vi "George_Illumination.vi"(0 "File Path":path=path "C:/Test_Data/George_Illumination/L127Capture Image_.bmp", 7 "error in":errorcluster) -> (20 "Line Profile (Illumination Line Profile [Horizantal])":cluster{"x0":sgl, "dx":sgl, "Pixels Line":sgl[]}={"x0"=0.0, "dx"=1.0, "Pixels Line"=[0.0]} {"Pixels Line" format="%.2f"; "dx" format="%.2f"; "x0" format="%.2f"}, 21 "ROI Pixel Statistics (Illumination Line Profile [Horizantal])":T2 {"Min" format="%.2f"; "Std Dev" format="%.2f"; "Mean" format="%.2f"; "Max" format="%.2f"}, 22 "Line Profile (Illumination Line Profile [Vertical])":cluster{"x0":sgl, "dx":sgl, "Pixels Line":sgl[]}={"x0"=0.0, "dx"=1.0, "Pixels Line"=[0.0]} {"Pixels Line" format="%.2f"; "dx" format="%.2f"; "x0" format="%.2f"}, 23 "ROI Pixel Statistics (Illumination Line Profile [Vertical])":T2 {"Min" format="%.2f"; "Std Dev" format="%.2f"; "Mean" format="%.2f"; "Max" format="%.2f"}, 27 "error out":errorcluster={"status"=TRUE, "code"=-1074396120, "source"="IMAQ ROIProfile\n  "})   [LabVIEW 2014]
uses:
  <vilib>/vision/NI_Vision_Development_Module.lvlib
panel:
  out "Image Out":T1(plugin-control)
  out "Line Profile Graph 2":cluster{"x0":sgl, "dx":sgl, "Pixels Line":sgl[]}(graph)={"x0"=0.0, "dx"=1.0, "Pixels Line"=[0.0]} caption="Line Profile"
  out "Line Profile Graph":cluster{"x0":sgl, "dx":sgl, "Pixels Line":sgl[]}(graph)={"x0"=0.0, "dx"=1.0, "Pixels Line"=[0.0]} caption="Line Profile"
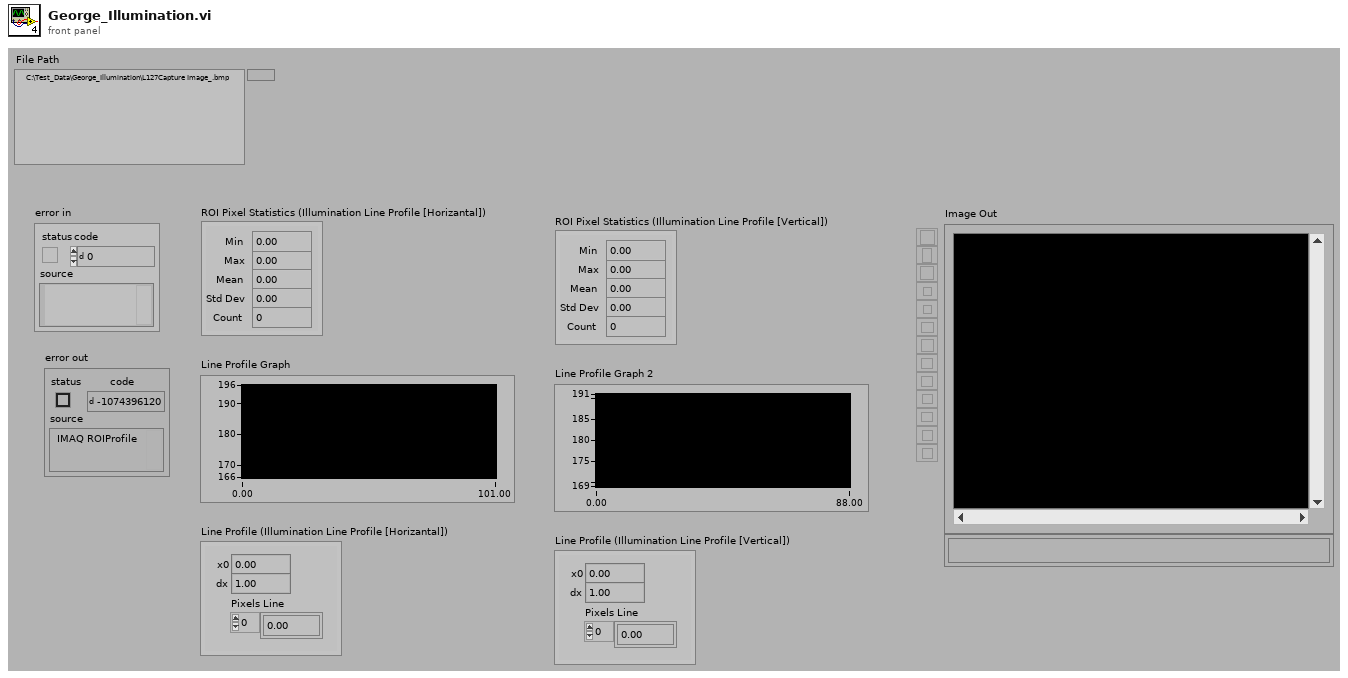
[diagram p1: front panel]
types:
  T1 = typedef "IMAQ Image.ctl" = refnum<image>
  T2 = cluster{"Min":sgl, "Max":sgl, "Mean":sgl, "Std Dev":sgl, "Count":i32}
  T3 = cluster{"Global Rectangle":i32[], "Contours":cluster{"ID":enum32{"External", "Internal"}, "Type":u32, "Coordinates":i32[]}[]}
  T4 = cluster{"Origin":cluster{"X":sgl, "Y":sgl}, "Angle (deg)":sgl, "Axis Reference":u32}
  T5 = enum16{"Reset", "Update Coordinate System", "Get Coordinate System"}
  T6 = enum16{"Horizontal Motion", "Vertical Motion", "Horizontal and Vertical Motion", "Horizontal, Vertical and Angular Motion"}
  T7 = typedef "Image Type" = u32
  T8 = typedef "IMAQ Coordinate System" = cluster{"Reference System":cluster{"Origin":cluster{"X":sgl, "Y":sgl}, "Angle (deg)":sgl, "Axis Reference":u32}, "Measurement System":cluster{"Origin":cluster{"X":sgl, "Y":sgl}, "Angle (deg)":sgl, "Axis Reference":u32}}
  T9 = typedef "ROI Descriptor" = cluster{"Global Rectangle":i32[], "Contours":cluster{"ID":enum32{"External", "Internal"}, "Type":u32, "Coordinates":i32[]}[]}
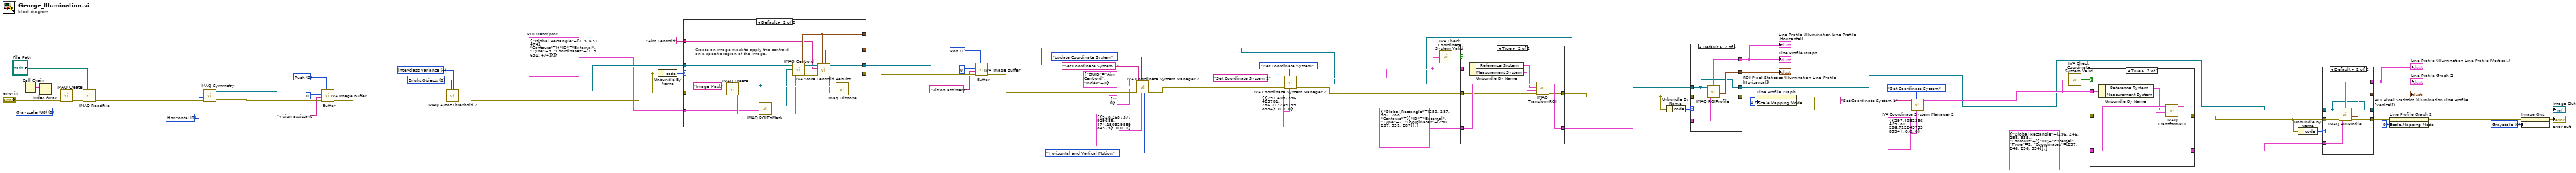
[diagram p0: block diagram]
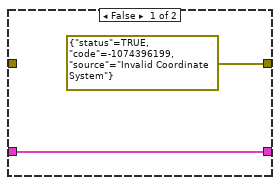
[diagram p3: hidden frame]
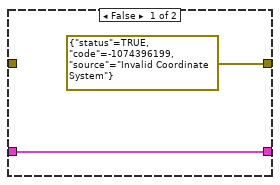
[diagram p5: hidden frame]
diagram:
  w3 = u32 0 items=["Grayscale", "Binary", "Gradient", "Rainbow", "Temperature", "User Defined"] ("Palette")
  w46 = u16 1 items=["Push", "Pop", "Reset"] ("Function")
  w51 = T3 {"Global Rectangle"=[7, 5, 631, 474], "Contours"=[{"ID"=enum."External", "Type"=3, "Coordinates"=[7, 5, 631, 474]}]}  # ROI Descriptor
  w54 = 4 items=["clustering", "entropy", "metric", "moments", "inter-class variance"] ("Method")
  w55 = u32 0 items=["Bright Objects", "Dark Objects"] ("Look For")
  w60 = u16 0 items=["Push", "Pop", "Reset"] ("Function")
  w63 = u32 0 items=["Horizontal", "Vertical", "Central", "1st Diagonal", "2nd Diagonal"] ("Type of Symmetry")
  w66 = T7 0 items=["Grayscale (U8)", "Grayscale (I16)", "Grayscale (SGL)", "Complex (CSG)", "RGB (U32)", "HSL (U32)", "RGB (U64)", "Grayscale (U16)"] ("Image Type")
  # "Buffer"
  # "Buffer"
  n1 = Call Chain() -> (call chain=w68:string[])
  n2 = Index Array(array=w68) -> (element=w67:string)  [unwired: 1 in]
  n3 = call "IMAQ Create"("Image Name"=w67, "Image Type"=w66, "error in (no error)"="error in") -> ("New Image"=w71:T1, "error out"=w70:errorcluster)  [unwired: 1 in, 1 out]
  n4 = call "IMAQ ReadFile"("File Path"="File Path", "error in (no error)"=w70, "Image"=w71) -> ("error out"=w72:errorcluster, "Image Out"=w65:T1)  [unwired: 2 in, 5 out]
  n5 = call "IMAQ Symmetry"("error in (no error)"=w72, "Type of Symmetry"=w63, "Image Src"=w65) -> ("error out"=w64:errorcluster, "Image Dst Out"=w62:T1)  [unwired: 1 in, 1 out]
  n6 = call <vilib>:"IVA Image Buffer.vi"("Function"=w60, "error in (no error)"=w64, "Prefix"="vision assistant", "Buffer #"=0, "Image In"=w62) -> ("error out"=w61:errorcluster, "Image Out"=w57:T1)  [unwired: 5 out]
  n7 = call "IMAQ AutoBThreshold 2"("Image Src"=w57, "Look For (Bright Objects)"=w55, "Method (clustering)"=w54, "error in (no error)"=w61) -> ("Image Dst Out"=w52:T1, "error out"=w56:errorcluster)  [unwired: 4 in, 6 out]
  n8 = Unbundle By Name(w56) -> ("code"=w49:i32)
  n9 = case shown="Default" w49 {
    tunnel: w56 -> [_ w84]
    tunnel: [_ w83] -> w53
    tunnel: w52 -> [w73 w81]
    tunnel: [w73 w80] -> w48
    tunnel: [_ w79] -> _
    tunnel: [_ w78] -> _
    tunnel: w51 -> [_ w77]
    tunnel: "Aim Centroid" ("Step Name") -> [_ w74]
    frame -1074396199, -1074396198 {
      # "Discard Coordinate System Error"
    }
    frame Default {
      # "Create an image mask to apply the centroid\non a specific region of the image."
      n10 = call "IMAQ Create"("Image Name"="Image Mask", "error in (no error)"=w84) -> ("New Image"=w87:T1, "error out"=w86:errorcluster)  [unwired: 2 in, 1 out]
      n11 = call "IMAQ ROIToMask"("error in (no error)"=w86, "ROI Descriptor"=w77, "Image"=w87) -> ("error out"=w82:errorcluster, "Image Out"=w85:T1)  [unwired: 2 in, 2 out]
      n12 = call "IMAQ Centroid"("error in (no error)"=w82, "Image Mask"=w85, "Image"=w81) -> ("error out"=w76:errorcluster, "Centroid"=w79:cluster{"X Centroid":sgl, "Y Centroid":sgl})  [unwired: 1 out]
      n13 = call <vilib>:"IVA Store Centroid Results.vi"("Centroid in"=w79, "error in (no error)"=w76, "Step Name"=w74, "Image in"=w81) -> ("error out"=w75:errorcluster, "Image dup"=w80:T1, "Calibrated Centroid"=w78:cluster{"X":sgl, "Y":sgl})  [unwired: 5 out]
      n14 = call "Imaq Dispose"("Image"=w87, "error in (no error)"=w75) -> ("error out"=w83:errorcluster)  [unwired: 1 in, 3 out]
    }
  }
  n15 = call <vilib>:"IVA Image Buffer.vi"("Function"=w46, "error in (no error)"=w53, "Prefix"="vision assistant", "Buffer #"=0, "Image In"=w48) -> ("error out"=w47:errorcluster, "Image Out"=w24:T1)  [unwired: 5 out]
  n16 = call <vilib>:"IVA Coordinate System Manager 2.vi"("Mode"=T6."Horizontal and Vertical Motion", "Reference System"=T4 {"Origin"={"X"=528.26874, "Y"=474.15033}, "Angle (deg)"=0.0, "Axis Reference"=0}, "Function"=T5."Update Coordinate System", "error in (no error)"=w47, "Angle ID"=cluster{"GUID":string, "Index":i32} {"GUID"="", "Index"=0}, "Origin ID"=cluster{"GUID":string, "Index":i32} {"GUID"="Aim Centroid", "Index"=0}, "Coordinate System Name"="Set Coordinate System 1") -> ("error out"=w37:errorcluster)  [unwired: 4 out]
  n17 = call <vilib>:"IVA Coordinate System Manager 2.vi"("Reference System"=T4 {"Origin"={"X"=297.40823, "Y"=286.71225}, "Angle (deg)"=0.0, "Axis Reference"=0}, "Function"=T5."Get Coordinate System", "error in (no error)"=w37, "Coordinate System Name"="Set Coordinate System 1") -> ("error out"=w34:errorcluster, "Coordinate System Out"=w30:T8)  [unwired: 3 in, 3 out]
  n18 = call <vilib>:"IVA Check Coordinate System Valid.vi"("Coordinate System"=w30) -> ("Valid?"=w29:bool)
  n19 = case shown="True" w29 {
    tunnel: T3 {"Global Rectangle"=[250, 287, 352, 288], "Contours"=[{"ID"=enum."External", "Type"=2, "Coordinates"=[250, 287, 351, 287]}]} ("ROI Descriptor") -> [w89 w97]
    tunnel: [w89 w94] -> w22
    tunnel: [errorcluster {"status"=TRUE, "code"=-1074396199, "source"="Invalid Coordinate System"} ("error out") w93] -> w31
    tunnel: w30 -> [_ w92]
    tunnel: w34 -> [_ w91]
    frame False {
    }
    frame True {
      n20 = Unbundle By Name(w92) -> ("Reference System"=w96:T4, "Measurement System"=w95:T4)
      n21 = call "IMAQ TransformROI"("error in (no error)"=w91, "New Reference"=w95, "Base Reference"=w96, "ROI Descriptor"=w97) -> ("error out"=w93:errorcluster, "ROI Descriptor out"=w94:T9)  [unwired: 6 out]
    }
  }
  n22 = Unbundle By Name(w31) -> ("code"=w21:i32)
  n23 = case shown="Default" w21 {
    tunnel: w31 -> [_ w104]
    tunnel: [_ w103] -> w28
    tunnel: [_ w102] -> w26
    tunnel: w24 -> [w98 w99]
    tunnel: [_ w101] -> w23
    tunnel: w22 -> [_ w100]
    tunnel: [w98 w99] -> w8
    frame -1074396199, -1074396198 {
      # "Discard\nCoordinate\nSystem\nError"
    }
    frame Default {
      n24 = call "IMAQ ROIProfile"("error in (no error)"=w104, "ROI Descriptor"=w100, "Image"=w99) -> ("ROI Pixel Statistics"=w103:T2, "error out"=w102:errorcluster, "ROI Graph"=w101:cluster{"x0":sgl, "dx":sgl, "Pixels Line":sgl[]})  [unwired: 3 out]
    }
  }
  "ROI Pixel Statistics (Illumination Line Profile [Horizantal])" <- w28
  "Line Profile Graph" <- w23
  "Line Profile (Illumination Line Profile [Horizantal])" <- w23
  n25 = property on="Line Profile Graph" class="WFGraph (strict)"(error in=w26, "Y Scale.Mapping Mode"=u8 0) -> (error out=w25:errorcluster)  [unwired: 1 in, 1 out]
  n26 = call <vilib>:"IVA Coordinate System Manager 2.vi"("Reference System"=T4 {"Origin"={"X"=297.40823, "Y"=286.71225}, "Angle (deg)"=0.0, "Axis Reference"=0}, "Function"=T5."Get Coordinate System", "error in (no error)"=w25, "Coordinate System Name"="Set Coordinate System 1") -> ("error out"=w18:errorcluster, "Coordinate System Out"=w14:T8)  [unwired: 3 in, 3 out]
  n27 = call <vilib>:"IVA Check Coordinate System Valid.vi"("Coordinate System"=w14) -> ("Valid?"=w13:bool)
  n28 = case shown="True" w13 {
    tunnel: T3 {"Global Rectangle"=[296, 246, 298, 335], "Contours"=[{"ID"=enum."External", "Type"=2, "Coordinates"=[297, 246, 296, 334]}]} ("ROI Descriptor") -> [w105 w113]
    tunnel: [w105 w110] -> w6
    tunnel: [errorcluster {"status"=TRUE, "code"=-1074396199, "source"="Invalid Coordinate System"} ("error out") w109] -> w15
    tunnel: w14 -> [_ w108]
    tunnel: w18 -> [_ w107]
    frame False {
    }
    frame True {
      n29 = Unbundle By Name(w108) -> ("Reference System"=w112:T4, "Measurement System"=w111:T4)
      n30 = call "IMAQ TransformROI"("error in (no error)"=w107, "New Reference"=w111, "Base Reference"=w112, "ROI Descriptor"=w113) -> ("error out"=w109:errorcluster, "ROI Descriptor out"=w110:T9)  [unwired: 6 out]
    }
  }
  n31 = Unbundle By Name(w15) -> ("code"=w5:i32)
  n32 = case shown="Default" w5 {
    tunnel: w15 -> [_ w120]
    tunnel: [_ w119] -> w12
    tunnel: [_ w118] -> w10
    tunnel: w8 -> [w114 w115]
    tunnel: [_ w117] -> w7
    tunnel: w6 -> [_ w116]
    tunnel: [w114 w115] -> w4
    frame -1074396199, -1074396198 {
      # "Discard\nCoordinate\nSystem\nError"
    }
    frame Default {
      n33 = call "IMAQ ROIProfile"("error in (no error)"=w120, "ROI Descriptor"=w116, "Image"=w115) -> ("ROI Pixel Statistics"=w119:T2, "error out"=w118:errorcluster, "ROI Graph"=w117:cluster{"x0":sgl, "dx":sgl, "Pixels Line":sgl[]})  [unwired: 3 out]
    }
  }
  "ROI Pixel Statistics (Illumination Line Profile [Vertical])" <- w12
  "Line Profile Graph 2" <- w7
  "Line Profile (Illumination Line Profile [Vertical])" <- w7
  "Image Out" <- w4
  n34 = property on="Line Profile Graph 2" class="WFGraph (strict)"(error in=w10, "Y Scale.Mapping Mode"=u8 0) -> (error out=w9:errorcluster)  [unwired: 1 in, 1 out]
  n35 = property on="Image Out" class="ImageControl"(error in=w9, "Palette:Palette Type"=w3) -> (error out=→"error out":errorcluster)  [unwired: 1 in, 1 out]
